vi "2021_day6_task1.vi"() -> ()   [LabVIEW 2021]
panel:
  out "Arr to overflow":i32
  out "Iteration":i32
  out "# of fish(s)":i32
  in  "# of Iteration":i32=265
  out "Input Data":i8[](array[numeric])
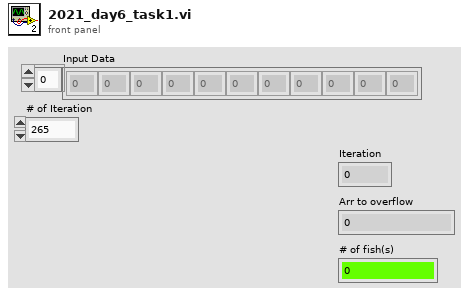
[diagram p1: front panel]
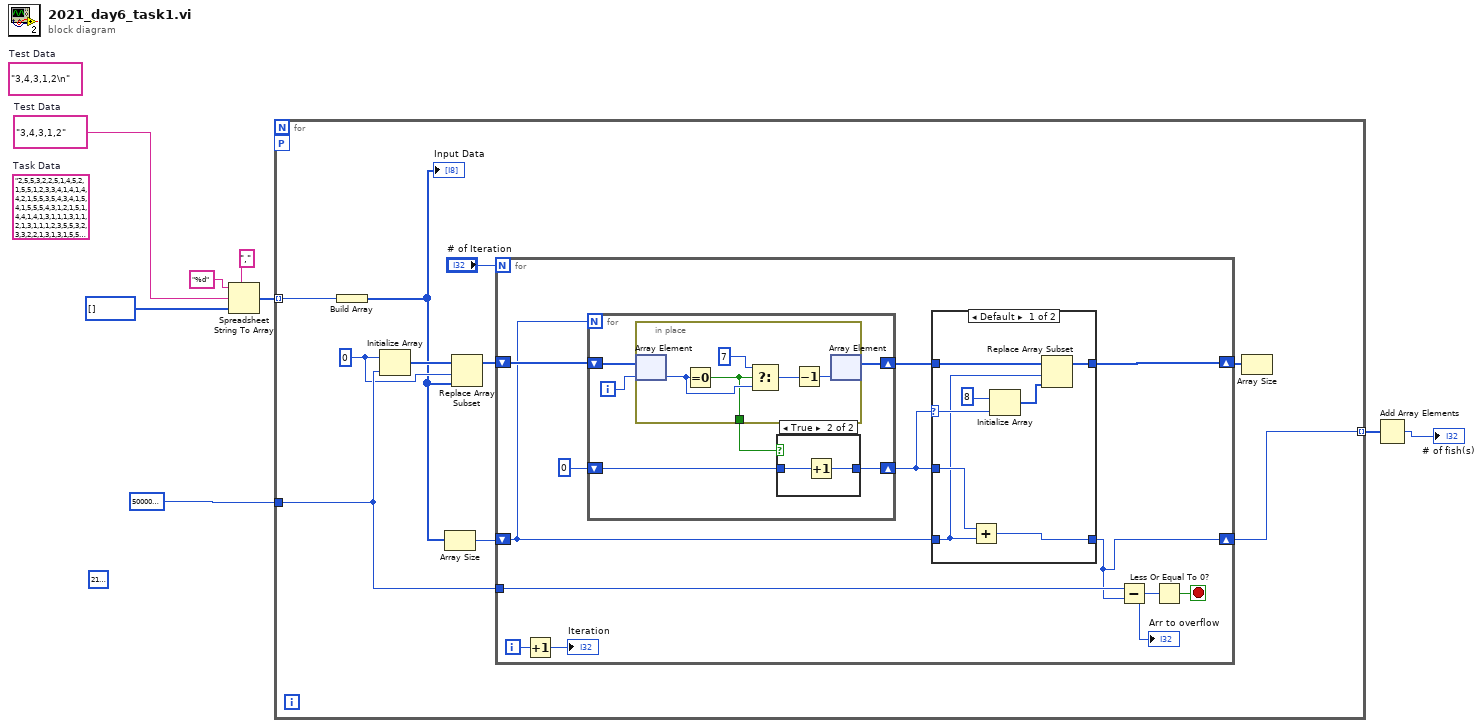
[diagram p0: block diagram]
diagram:
  (unwired) "3,4,3,1,2\n"  # Test Data
  (unwired) 2147483647
  (unwired) "2,5,5,3,2,2,5,1,4,5,2,1,5,5,1,2,3,3,4,1,4,1,4,4,2,1,5,5,3,5,4,3,4,1,5,4,1,5,5,5,4,3,1,2,1,5,1,4,4,1,4,1,3,1,1,1,3,1,1,2,1,3,1,1,1,2,3,5,5,3,2,3,3,2,2,1,3,1,3,1,5,5,1,2,3,2,1,1,2,1,2,1,2,2,1,3,5,4,3,3,2,2,3,1,4,2,2,1,3,4,5,4,2,5,4,1,2,1,3,5,3,3,5,4,1,1,5,2,4,4,1,2,2,5,5,3,1,2,4,3,3,1,4,2,5,1,5,1,2,1,1,1,1,3,5,5,1,5,5,1,2,2,1,2,1,2,1,2,1,4,5,1,2,4,3,3,3,1,5,3,2,2,1,4,2,4,2,3,2,5,1,5,1,1,1,3,1,1,3,5,4,2,5,3,2,2,1,4,5,1,3,2,5,1,2,1,4,1,5,5,1,2,2,1,2,4,5,3,3,1,4,4,3,1,4,2,4,4,3,4,1,4,5,3,1,4,2,2,3,4,4,4,1,4,3,1,3,4,5,1,5,4,4,4,5,5,5,2,1,3,4,3,2,5,3,1,3,2,2,3,1,4,5,3,5,5,3,2,3,1,2,5,2,1,3,1,1,1,5,1"  # Task Data
  w3 = "3,4,3,1,2"  # Test Data
  n1 = Spreadsheet String To Array(delimiter (Tab)=",", format string="%d", spreadsheet string=w3, array type (2D Dbl)=i8[] []) -> (array=w4:i8[])
  n2 = for {
    tunnel: 500000000 -> [w16]
    tunnel: w4 -> [w14] mode=indexing
    tunnel: [w9] -> w2 mode=indexing
    workers-P: _ -> [_]
    w12 = i8 0
    n3 = Build Array(w14) -> (w10:i8[])
    "Input Data" <- w10
    n4 = Initialize Array(w12, w16) -> (w15:i8[])
    n5 = Array Size(array=w10) -> (size(s)=w11:i32)
    n6 = Replace Array Subset(array=w15, new element=w10, index=w12) -> (w13:i8[])
    n7 = for {
      N: "# of Iteration" -> [_]
      shift-right: [w24] -> w17
      shift-left: w13 -> [w26]
      shift-right: [w22] -> w9
      shift-left: w11 -> [w21]
      tunnel: w16 -> [w28]
      i -> [w29]
      stop <- w27 stop-if-true
      n8 = Increment(x=w29) -> (x+1=→"Iteration":i32)
      n9 = for {
        N: w21 -> [_]
        shift-right: [w44] -> w30
        shift-left: w26 -> [w46]
        shift-right: [w42] -> w23
        shift-left: 0 -> [w43]
        i -> [w45]
        n10 = in-place {
          in-place-border: [w51] -> w41
          n11 = in-place-array #1(w46, w45) -> (w52:i8)
          n12 = Equal To 0?(x=w52) -> (x = 0?=w51:bool)
          n13 = Select(t=i8 7, s=w51, f=w52) -> (s? t:f=w53:i8)
          n14 = Decrement(x=w53) -> (x-1=w50:i8)
          n15 = in-place-array #1(w50) -> (w44:i8[])  [unwired: 1 out]
        }
        n16 = case shown="True" w41 {
          tunnel: w43 -> [w47 w49]
          tunnel: [w47 w48] -> w42
          frame False {
          }
          frame True {
            n17 = Increment(x=w49) -> (x+1=w48:i32)
          }
        }
      }
      n18 = case shown="Default" w23 {
        selector: w23 -> [w35 _]
        tunnel: w30 -> [w38 w40]
        tunnel: [w37 w40] -> w24
        tunnel: w23 -> [w33 _]
        tunnel: w21 -> [w31 w39]
        tunnel: [w32 w39] -> w22
        frame Default {
          n19 = Add(x=w33, y=w31) -> (x+y=w32:i32)
          n20 = Initialize Array(i8 8, w35) -> (w36:i8[])
          n21 = Replace Array Subset(array=w38, new element=w36, index=w31) -> (w37:i8[])
        }
        frame 0 {
        }
      }
      n22 = Subtract(x=w28, y=w22) -> (x-y=w20:i32)
      "Arr to overflow" <- w20
      n23 = Less Or Equal To 0?(x=w20) -> (x <= 0?=w27:bool)
    }
    n24 = Array Size(array=w17) -> ()  [unwired: 1 out]
  }
  n25 = Add Array Elements(numeric array=w2) -> (sum=→"# of fish(s)":i32)
